vi "graphDICH.vi"() -> ()   [LabVIEW 2019]
panel:
  in  "Y Scale.Range:Minimum":dbl
  in  "Y Scale.Range:Maximum":dbl
  in  "X Scale.Range:Minimum":dbl
  in  "X Scale.Range:Maximum":dbl
  out "XY Graph 2":cluster{"X":dbl, "Y":dbl}[](graph)
  out "XY Graph":cluster{"X":dbl, "Y":dbl}[](graph)
  in  "stop":bool
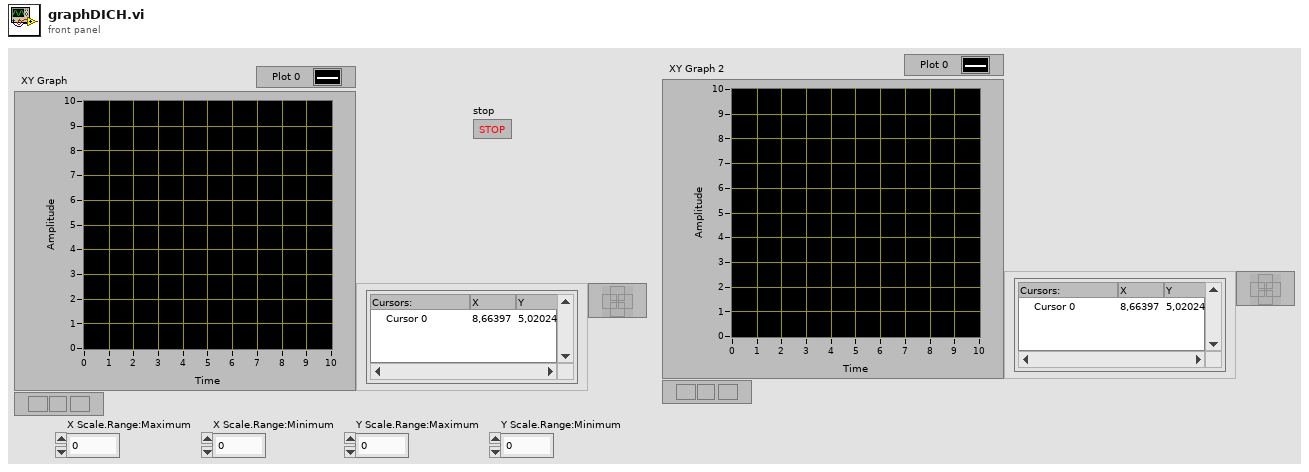
[diagram p1: front panel]
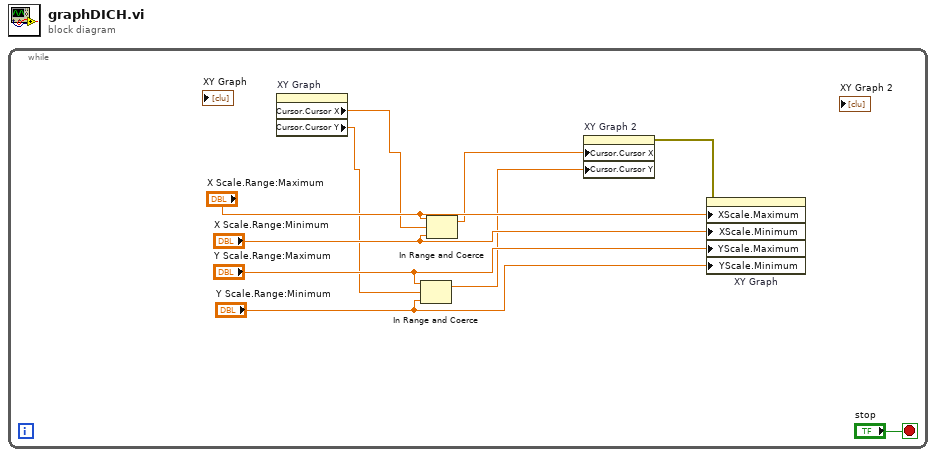
[diagram p0: block diagram]
diagram:
  n1 = while {
    stop <- "stop" stop-if-true
    n2 = property on="XY Graph" class="XYGraph (strict)"() -> ("Cursor.Cursor X"=w6:dbl, "Cursor.Cursor Y"=w2:dbl)  [unwired: 2 in, 2 out]
    n3 = In Range and Coerce(upper limit="Y Scale.Range:Maximum", x=w2, lower limit="Y Scale.Range:Minimum") -> (coerced(x)=w1:dbl)  [unwired: 1 out]
    n4 = In Range and Coerce(upper limit="X Scale.Range:Maximum", x=w6, lower limit="X Scale.Range:Minimum") -> (coerced(x)=w5:dbl)  [unwired: 1 out]
    n5 = property on="XY Graph 2" class="XYGraph (strict)"("Cursor.Cursor X"=w5, "Cursor.Cursor Y"=w1) -> (error out=w9:errorcluster)  [unwired: 2 in, 1 out]
    n6 = property on="XY Graph" class="XYGraph (strict)"(error in=w9, "XScale.Maximum"="X Scale.Range:Maximum", "XScale.Minimum"="X Scale.Range:Minimum", "YScale.Maximum"="Y Scale.Range:Maximum", "YScale.Minimum"="Y Scale.Range:Minimum") -> ()  [unwired: 1 in, 2 out]
  }
